vi "Wait For Bytes.vi"(8 "Error In":errorcluster, 9 "Time Out (100 ms)":i32=1000, 10 "Bytes To Read":u32, 11 "VISA resource name":refnum<visa-resource-name>) -> (0 "Error Out":errorcluster, 2 "Bytes Available?":bool, 3 "VISA resource name":refnum<visa-resource-name>)   [LabVIEW 2011, in "LVH-EZ430.lvlib"]
doc: "Wait for the specified number of bytes to be available in the VISA buffer."
uses:
  <vilib>/LabVIEW Hacker/LabVIEW Interface for EZ430-Chronos/LVH-EZ430.lvlib
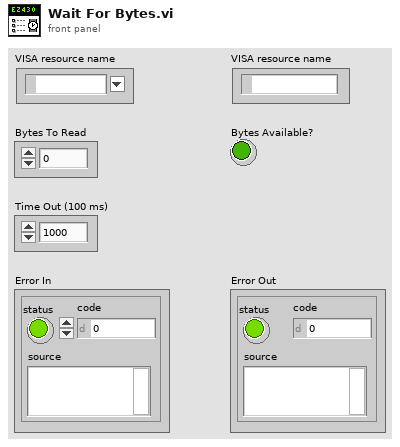
[diagram p1: front panel]
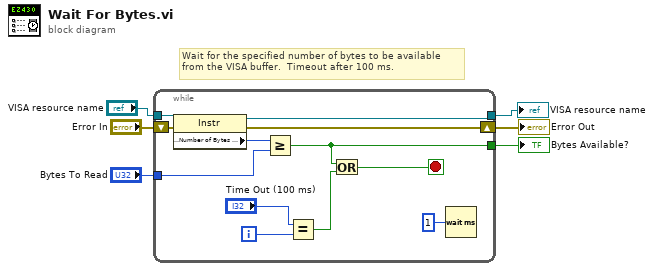
[diagram p0: block diagram]
diagram:
  # "Wait for the specified number of bytes to be available\nfrom the VISA buffer.  Timeout after 100 ms."
  n1 = while {
    tunnel: "Bytes To Read" -> [w11]
    tunnel: [w18] -> w1
    tunnel: "VISA resource name" -> [w14]
    shift-right: [w10] -> w4
    shift-left: "Error In" -> [w13]
    tunnel: [w7] -> w3
    i -> [w16]
    stop <- w8 stop-if-true
    n2 = property class="Instr"(reference=w14, error in=w13) -> (reference out=w18:refnum<visa-resource-name>, error out=w10:errorcluster, "Serial Settings:Number of Bytes at Serial Port"=w12:u32)
    n3 = Greater Or Equal?(x=w12, y=w11) -> (x >= y?=w7:bool)
    n4 = Equal?(x="Time Out (100 ms)", y=w16) -> (x = y?=w9:bool)
    n5 = Or(x=w7, y=w9) -> (x .or. y?=w8:bool)
    n6 = Wait (ms)(milliseconds to wait=u32 1) -> ()  [unwired: 1 out]
  }
  "Error Out" <- w4
  "Bytes Available?" <- w3
  "VISA resource name" <- w1
